vi "SUB_SearchFile_inAnyFolder.vi"(4 "Search Filename in Folder":string, 5 "Base path":string) -> (0 "TARGET PATH":path, 1 "spreadsheet string":string, 2 "File Existing True/Flase":bool)   [LabVIEW 2011]
panel:
  out "error out":errorcluster
  out "string":string
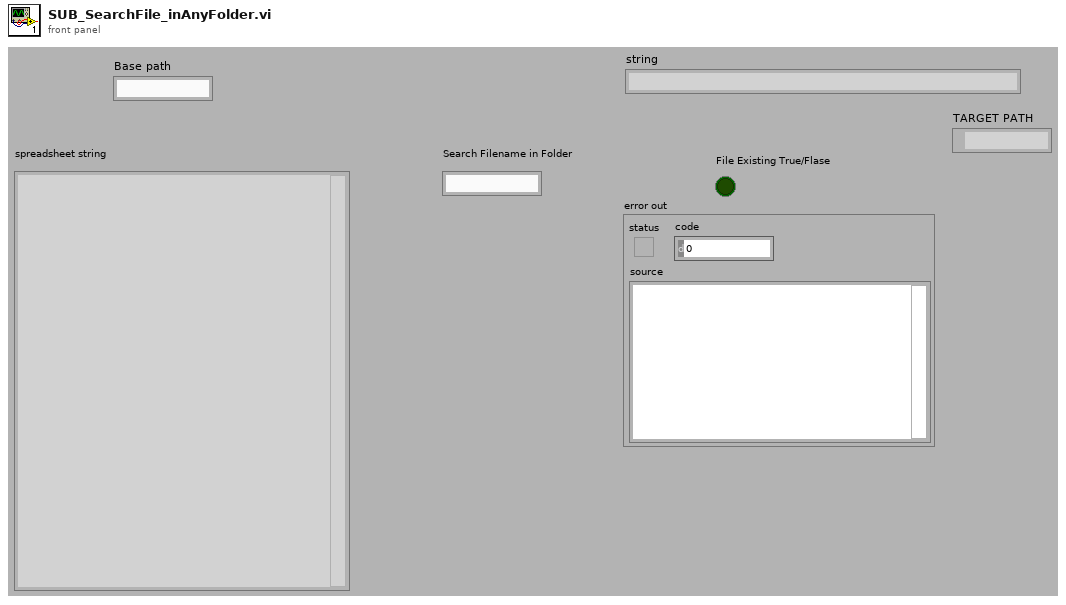
[diagram p1: front panel]
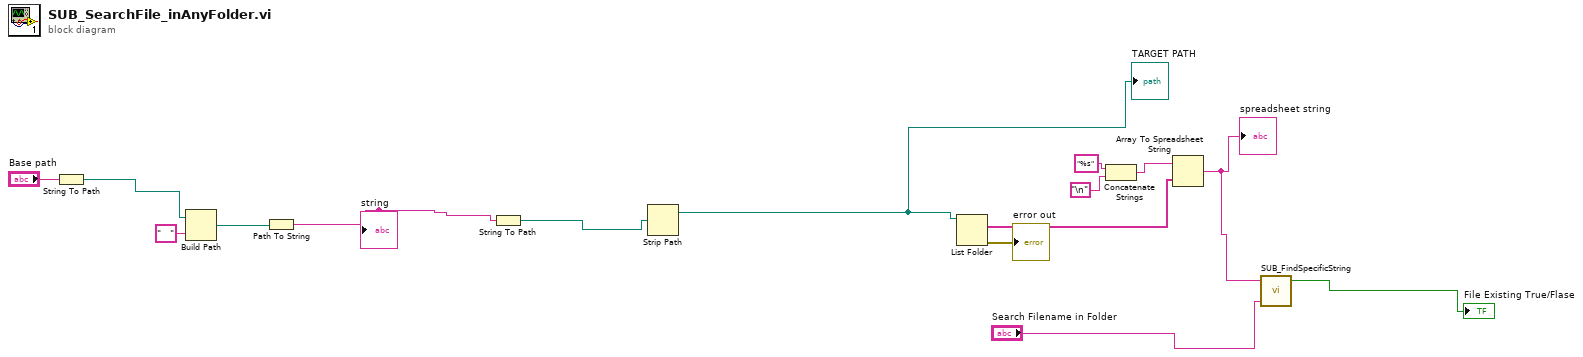
[diagram p0: block diagram]
diagram:
  n1 = String To Path(string="Base path") -> (path=w5:path)
  n2 = Build Path(base path=w5, name or relative path="   ") -> (appended path=w11:path)
  n3 = Path To String(path=w11) -> (string=w10:string)
  "string" <- w10
  n4 = String To Path(string=w10) -> (path=w2:path)
  n5 = Strip Path(path=w2) -> (stripped path=w1:path)  [unwired: 1 out]
  "TARGET PATH" <- w1
  n6 = List Folder(path=w1) -> (filenames=w15:string[], error out=→"error out":errorcluster)  [unwired: 3 in, 2 out]
  n7 = Concatenate Strings("%s" ("format string"), "\n") -> (w12:string)
  n8 = Array To Spreadsheet String(array=w15, 3:w12) -> (spreadsheet string=w8:string)  [unwired: 1 in]
  "spreadsheet string" <- w8
  n9 = call "SUB_FindSpecificString.vi"("Find this String"="Search Filename in Folder", "String data"=w8) -> ("Found"=→"File Existing True/Flase":bool)  [unwired: 2 in, 1 out]
